vi "_main__.vi"() -> ()   [LabVIEW 2015]
doc: "Dialtek PKT-8 test programm"
uses:
  <vilib>/NI/Modbus Library/API/Master/Modbus Master.lvclass
  Load and Save Controls_LV2009.llb/RWC_Actions.ctl
  <vilib>/Utility/error.llb/DialogType.ctl
panel:
  out "Связь с блоком":bool
  in  "счетчик":u16
  in  "Tab Control":enum32{"Измерения", "Коэффициенты", "Настройки"}(tab)
  out "R8":dbl format="%.2f"
  out "R7":dbl format="%.2f"
  out "R6":dbl format="%.2f"
  out "R5":dbl format="%.2f"
  out "R4":dbl format="%.2f"
  out "R3":dbl format="%.2f"
  out "R2":dbl format="%.2f"
  out "R1":dbl format="%.2f"
  in  "8_ch_visible":bool=TRUE
  out "8":dbl format="%.2f"
  out "7":dbl format="%.2f"
  in  "7_ch_visible":bool=TRUE
  out "6":dbl format="%.2f"
  in  "6_ch_visible":bool=TRUE
  out "5":dbl format="%.2f"
  in  "5_ch_visible":bool=TRUE
  in  "4_ch_visible":bool=TRUE
  out "4":dbl format="%.2f"
  in  "3_ch_visible":bool=TRUE
  out "3":dbl format="%.2f"
  in  "2_ch_visible":bool=TRUE
  out "2":dbl format="%.2f"
  in  "1_ch_visible":bool=TRUE
  out "1":dbl format="%.2f"
  in  "xScale -":bool
  in  "xScale +":bool
  out "мин.":string="1"
  in  "Добавить время":dbl(ring)=300.0 items=["10 сек."=10.0, "1 мин."=60.0, "5 мин."=300.0, "20 мин."=1200.0]
  out "часы":string="0"
  out "сек.":string="0"
  in  "Coeff_cl_ch8":T1 caption="Канал 8" {"R" format="%#_16g"; "k7" format="%#_16g"; "k6" format="%#_16g"; "k5" format="%#_16g"; "k4" format="%#_16g"; "k3" format="%#_16g"; "k2" format="%#_16g"; "k1" format="%#_16g"}
  in  "Coeff_cl_ch7":T1 caption="Канал 7" {"R" format="%#_16g"; "k7" format="%#_16g"; "k6" format="%#_16g"; "k5" format="%#_16g"; "k4" format="%#_16g"; "k3" format="%#_16g"; "k2" format="%#_16g"; "k1" format="%#_16g"}
  in  "Coeff_cl_ch6":T1 caption="Канал 6" {"R" format="%#_16g"; "k7" format="%#_16g"; "k6" format="%#_16g"; "k5" format="%#_16g"; "k4" format="%#_16g"; "k3" format="%#_16g"; "k2" format="%#_16g"; "k1" format="%#_16g"}
  in  "Coeff_cl_ch5":T1 caption="Канал 5" {"R" format="%#_16g"; "k7" format="%#_16g"; "k6" format="%#_16g"; "k5" format="%#_16g"; "k4" format="%#_16g"; "k3" format="%#_16g"; "k2" format="%#_16g"; "k1" format="%#_16g"}
  in  "Coeff_cl_ch4":T1 caption="Канал 4" {"R" format="%#_16g"; "k7" format="%#_16g"; "k6" format="%#_16g"; "k5" format="%#_16g"; "k4" format="%#_16g"; "k3" format="%#_16g"; "k2" format="%#_16g"; "k1" format="%#_16g"}
  in  "Coeff_cl_ch3":T1 caption="Канал 3" {"R" format="%#_16g"; "k7" format="%#_16g"; "k6" format="%#_16g"; "k5" format="%#_16g"; "k4" format="%#_16g"; "k3" format="%#_16g"; "k2" format="%#_16g"; "k1" format="%#_16g"}
  in  "Coeff_cl_ch2":T1 caption="Канал 2" {"R" format="%#_16g"; "k7" format="%#_16g"; "k6" format="%#_16g"; "k5" format="%#_16g"; "k4" format="%#_16g"; "k3" format="%#_16g"; "k2" format="%#_16g"; "k1" format="%#_16g"}
  in  "Coeff_cl_ch1":T1 caption="Канал 1" {"R" format="%#_16g"; "k7" format="%#_16g"; "k6" format="%#_16g"; "k5" format="%#_16g"; "k4" format="%#_16g"; "k3" format="%#_16g"; "k2" format="%#_16g"; "k1" format="%#_16g"}
  in  "Сохранение в файл":bool=TRUE
  in  "интервал, сек.":u16=10 min=1 max=3600 step=1
  out "Path":string
  in  "buffer":u16=20 min=1 max=128
  in  "SPS":enum16{"2,5 SPS", "5 SPS", "10 SPS"}(ring)=enum."5 SPS"
  in  "ID":u8
  in  "Порт":u16
  in  "IP":string
  in  "Т min":dbl=4.0 min=-10.0 max=350.0 step=0.01
  in  "Т max":dbl=150.0 min=-10.0 max=150.0 step=0.01
  in  "Autoscale":bool=TRUE
  in  "Autoscale R":bool=TRUE
  in  "R max":dbl=150.0 min=-10.0 max=150.0 step=0.01
  in  "R min":dbl=4.0 min=-10.0 max=150.0 step=0.01
  out "refnum out":refnum<file>
  in  "stop":bool
  out "Сутки":string
  out "File header exist?":bool caption="Disconn"
  out "Graphs T":dynamicdata(graph) caption="T, K"
  out "Соед.":refnum<class "Modbus Master.lvclass">
  out "Graphs R":dynamicdata(graph) caption="R, Oм"
  # "№"
  # "T [ K ]"
  # "R [ Ohm ]"
  # ":"
  # ":"
  # "Настройки соединения"
  # "Настройки сохранения"
  # "Настройки АЦП"
  # "Буфер. усредн."
  # "Скорость изм."
  # "SPS = Samples Per Sec."
  # "Шкала Т"
  # "Шкала R"
types:
  T1 = cluster{"k1":ext, "k2":ext, "k3":ext, "k4":ext, "k5":ext, "k6":ext, "k7":ext, "R":ext}
  T2 = typedef "DialogType.ctl" = u16
  T3 = typedef "RWC_Actions.ctl" = enum16{"Read", "Write", "Read and Create"}
  T4 = typedef "LVDateTimeRec.ctl" = cluster{"fractional second":dbl, "second":i32, "minute":i32, "hour":i32, "day of month":i32, "month":i32, "year":i32, "day of week":i32, "day of year":i32, "DST":i32}
  T5 = cluster{"R1":dbl, "R2":dbl, "R3":dbl, "R4":dbl, "R5":dbl, "R6":dbl, "R7":dbl, "R8":dbl}
  T6 = cluster{"1":dbl, "2":dbl, "3":dbl, "4":dbl, "5":dbl, "6":dbl, "7":dbl, "8":dbl}
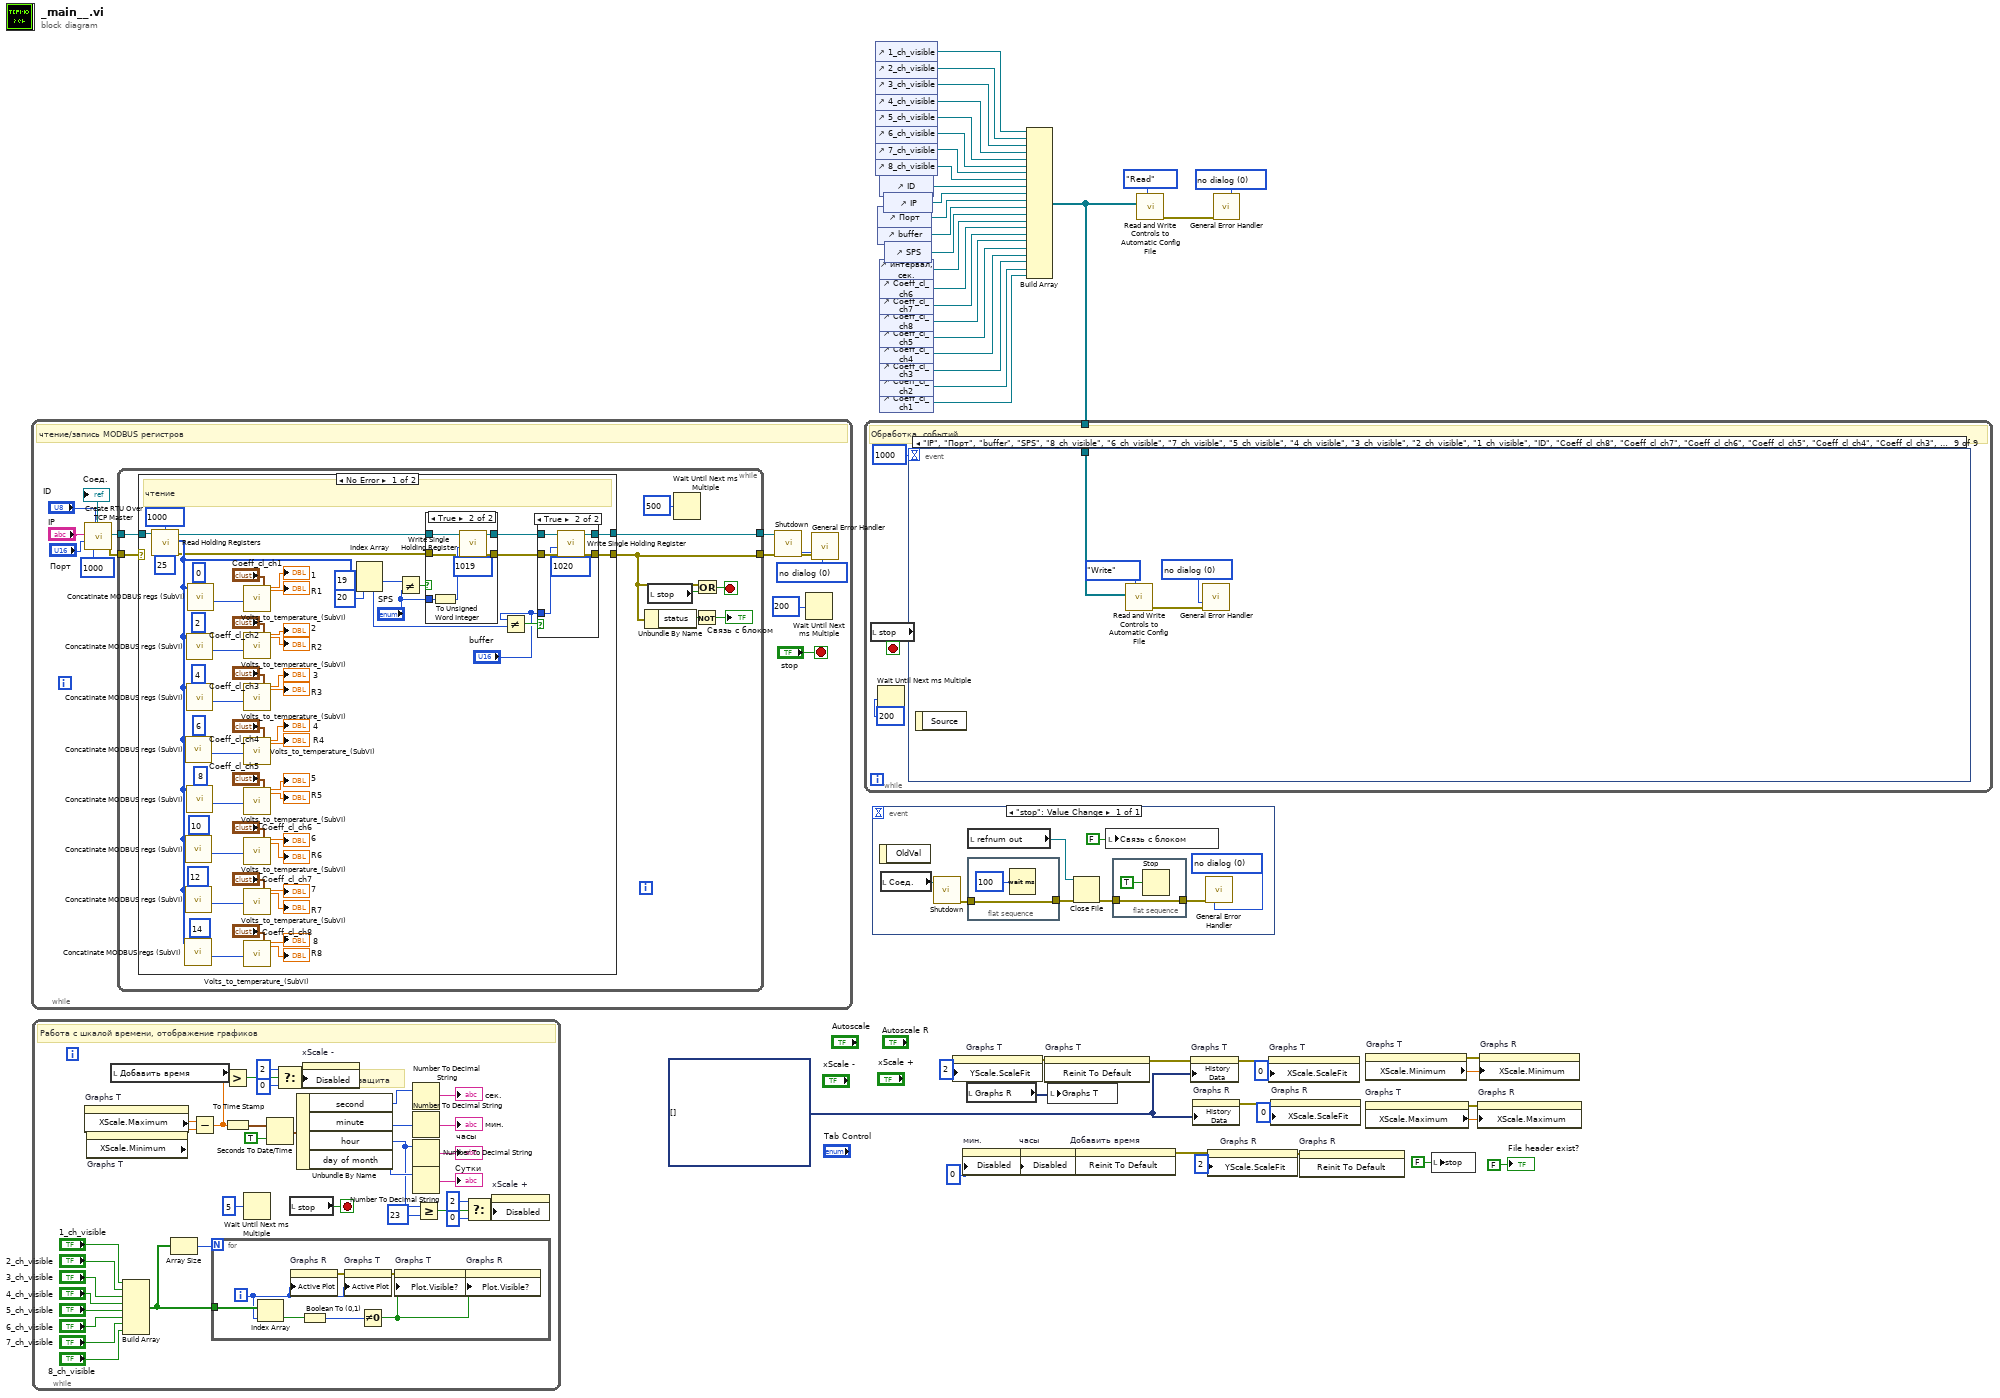
[diagram p0: block diagram]
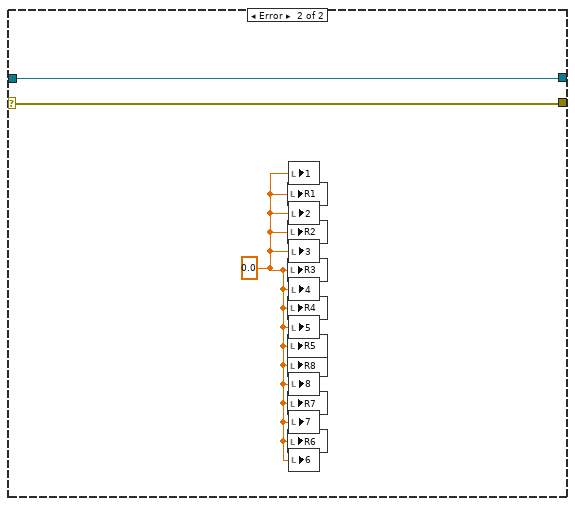
[diagram p4: hidden frame]
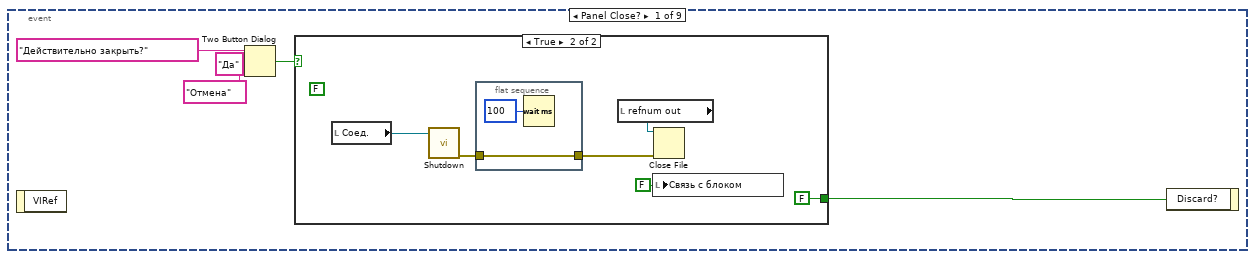
[diagram p5: hidden frame]
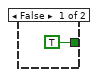
[diagram p6: hidden frame]
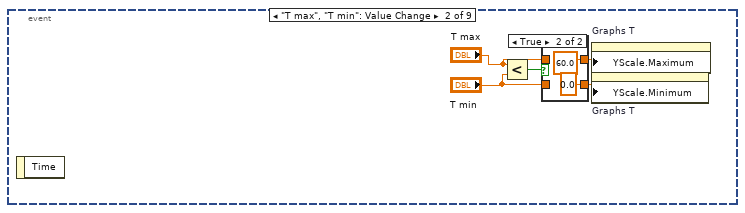
[diagram p7: hidden frame]
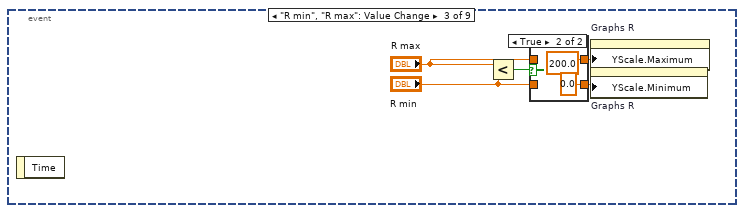
[diagram p9: hidden frame]
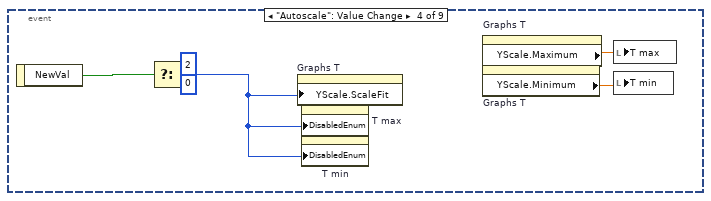
[diagram p11: hidden frame]
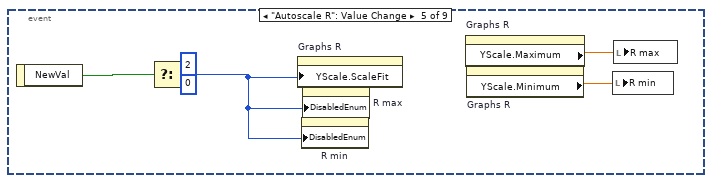
[diagram p12: hidden frame]
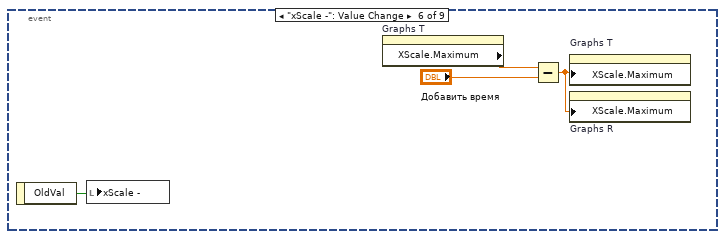
[diagram p13: hidden frame]
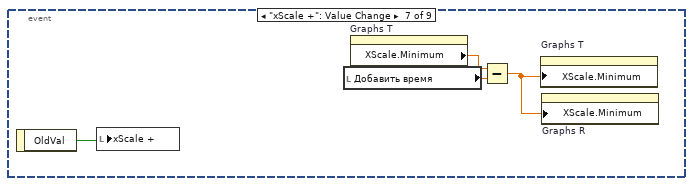
[diagram p14: hidden frame]
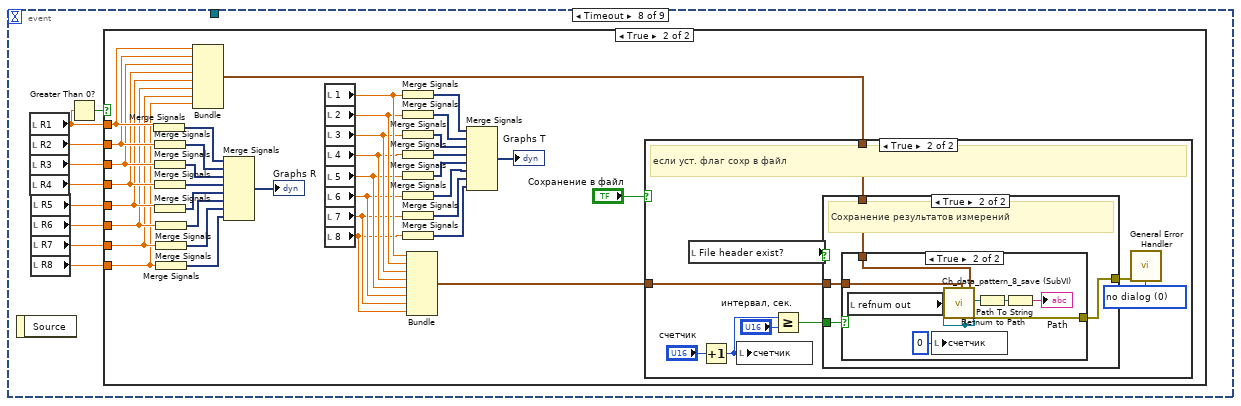
[diagram p15: hidden frame]
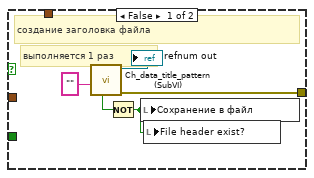
[diagram p18: hidden frame]
diagram:
  w13 = T2 0 items=["no dialog", "OK message", "continue or stop message", "OK message + warnings", "continue/stop + warnings"] ("type of dialog (OK msg:1)")
  w29 = dynamicdata[] [] ("History Data")
  w47 = u8 0 ("Disabled")
  n1 = while {
    stop <- "stop" stop-if-true
    w51 = T2 0 items=["no dialog", "OK message", "continue or stop message", "OK message + warnings", "continue/stop + warnings"] ("type of dialog (OK msg:1)")
    # "чтение/запись MODBUS регистров"
    n2 = call "Create RTU Over TCP Master.vi"("unit ID"="ID", "connect timeout ms"=1000, "port (502)"="Порт", "address"="IP") -> ("error out"=w55:errorcluster, "TCP master instance"=w56:refnum<class "Modbus Master.lvclass">)  [unwired: 6 in]
    "Соед." <- w56
    n3 = while {
      tunnel: w56 -> [w68]
      tunnel: w55 -> [w67]
      tunnel: [w61] -> w54
      tunnel: [w66] -> w53
      stop <- w64 stop-if-true
      n4 = case shown="No Error" w67 {
        selector: w67 -> [_ w145]
        tunnel: w68 -> [w124 w146]
        tunnel: [w103 w145] -> w61
        tunnel: [w104 w146] -> w66
        frame No Error {
          # "чтение"
          n5 = call-dynamic "Read Holding Registers.vi"("number of inputs"=u16 25, "starting address"=u16 1000, "Modbus master in"=w124) -> ("error out"=w102:errorcluster, "register values"=w106:u16[], "Modbus master out"=w107:refnum<class "Modbus Master.lvclass">)  [unwired: 6 in]
          n6 = call "Concatinate MODBUS regs (SubVI).vi"("LSB reg num"=u16 14, "registers array in"=w106) -> ("register data"=w81:i32)  [unwired: 8 in, 1 out]
          n7 = call "Concatinate MODBUS regs (SubVI).vi"("LSB reg num"=u16 6, "registers array in"=w106) -> ("register data"=w86:i32)  [unwired: 8 in, 1 out]
          n8 = call "Concatinate MODBUS regs (SubVI).vi"("LSB reg num"=u16 10, "registers array in"=w106) -> ("register data"=w83:i32)  [unwired: 8 in, 1 out]
          n9 = call "Concatinate MODBUS regs (SubVI).vi"("LSB reg num"=u16 12, "registers array in"=w106) -> ("register data"=w82:i32)  [unwired: 8 in, 1 out]
          n10 = call "Concatinate MODBUS regs (SubVI).vi"("LSB reg num"=u16 2, "registers array in"=w106) -> ("register data"=w95:i32)  [unwired: 8 in, 1 out]
          n11 = call "Concatinate MODBUS regs (SubVI).vi"("LSB reg num"=u16 4, "registers array in"=w106) -> ("register data"=w92:i32)  [unwired: 8 in, 1 out]
          n12 = call "Concatinate MODBUS regs (SubVI).vi"("LSB reg num"=u16 8, "registers array in"=w106) -> ("register data"=w84:i32)  [unwired: 8 in, 1 out]
          n13 = call "Concatinate MODBUS regs (SubVI).vi"("LSB reg num"=u16 0, "registers array in"=w106) -> ("register data"=w100:i32)  [unwired: 8 in, 1 out]
          n14 = call "Volts_to_temperature_(SubVI).vi"("input variable"=w100, "koeff. cluster"="Coeff_cl_ch1") -> ("T solvation"=→"1":dbl, "meas_voltage"=→"R1":dbl)  [unwired: 23 in, 1 out]
          n15 = call "Volts_to_temperature_(SubVI).vi"("input variable"=w95, "koeff. cluster"="Coeff_cl_ch2") -> ("T solvation"=→"2":dbl, "meas_voltage"=→"R2":dbl)  [unwired: 23 in, 1 out]
          n16 = call "Volts_to_temperature_(SubVI).vi"("input variable"=w92, "koeff. cluster"="Coeff_cl_ch3") -> ("T solvation"=→"3":dbl, "meas_voltage"=→"R3":dbl)  [unwired: 23 in, 1 out]
          n17 = call "Volts_to_temperature_(SubVI).vi"("input variable"=w86, "koeff. cluster"="Coeff_cl_ch4") -> ("T solvation"=→"4":dbl, "meas_voltage"=→"R4":dbl)  [unwired: 23 in, 1 out]
          n18 = call "Volts_to_temperature_(SubVI).vi"("input variable"=w84, "koeff. cluster"="Coeff_cl_ch5") -> ("T solvation"=→"5":dbl, "meas_voltage"=→"R5":dbl)  [unwired: 23 in, 1 out]
          n19 = call "Volts_to_temperature_(SubVI).vi"("input variable"=w83, "koeff. cluster"="Coeff_cl_ch6") -> ("T solvation"=→"6":dbl, "meas_voltage"=→"R6":dbl)  [unwired: 23 in, 1 out]
          n20 = call "Volts_to_temperature_(SubVI).vi"("input variable"=w82, "koeff. cluster"="Coeff_cl_ch7") -> ("T solvation"=→"7":dbl, "meas_voltage"=→"R7":dbl)  [unwired: 23 in, 1 out]
          n21 = call "Volts_to_temperature_(SubVI).vi"("input variable"=w81, "koeff. cluster"="Coeff_cl_ch8") -> ("T solvation"=→"8":dbl, "meas_voltage"=→"R8":dbl)  [unwired: 23 in, 1 out]
          n22 = Index Array(array=w106, index #1=19 ("index"), index #2=20 ("index")) -> (element #1=w110:u16, element #2=w115:u16)
          n23 = Not Equal?(x=w110, y="SPS") -> (x != y?=w111:bool)
          n24 = case shown="True" w111 {
            tunnel: w107 -> [w136 w143]
            tunnel: [w136 w141] -> w108
            tunnel: [w135 w140] -> w109
            tunnel: "SPS" -> [_ w138]
            tunnel: w102 -> [w135 w137]
            frame False {
            }
            frame True {
              n25 = To Unsigned Word Integer(number=w138) -> (unsigned 16bit integer=w139:u16)
              n26 = call-dynamic "Write Single Holding Register.vi"("error in"=w137, "register to write"=w139, "address"=u16 1019 ("starting address"), "Modbus master in"=w143) -> ("error out"=w140:errorcluster, "Modbus master out"=w141:refnum<class "Modbus Master.lvclass">)  [unwired: 6 in]
            }
          }
          n27 = Not Equal?(x="buffer", y=w115) -> (x != y?=w114:bool)
          n28 = case shown="True" w114 {
            tunnel: w108 -> [w128 w134]
            tunnel: w109 -> [w127 w133]
            tunnel: [w128 w131] -> w104
            tunnel: [w127 w130] -> w103
            tunnel: "buffer" -> [_ w129]
            frame False {
            }
            frame True {
              n29 = call-dynamic "Write Single Holding Register.vi"("error in"=w133, "register to write"=w129, "address"=u16 1020 ("starting address"), "Modbus master in"=w134) -> ("error out"=w130:errorcluster, "Modbus master out"=w131:refnum<class "Modbus Master.lvclass">)  [unwired: 6 in]
            }
          }
        }
        frame Error {
          w144 = 0.0 ("T1")
          n30 = local write "R1"(w144) -> ()
          n31 = local write "R2"(w144) -> ()
          n32 = local write "R3"(w144) -> ()
          n33 = local write "R4"(w144) -> ()
          n34 = local write "R5"(w144) -> ()
          n35 = local write "R8"(w144) -> ()
          n36 = local write "R7"(w144) -> ()
          n37 = local write "R6"(w144) -> ()
          n38 = local write "1"(w144) -> ()
          n39 = local write "2"(w144) -> ()
          n40 = local write "3"(w144) -> ()
          n41 = local write "4"(w144) -> ()
          n42 = local write "5"(w144) -> ()
          n43 = local write "8"(w144) -> ()
          n44 = local write "7"(w144) -> ()
          n45 = local write "6"(w144) -> ()
        }
      }
      n46 = Unbundle By Name(w61) -> ("status"=w63:bool)
      n47 = local read "stop"() -> (w65:bool)
      n48 = Wait Until Next ms Multiple(millisecond multiple=u32 500) -> ()  [unwired: 1 out]
      n49 = Not(x=w63) -> (.not. x?=→"Связь с блоком":bool)
      n50 = Or(x=w61, y=w65) -> (x .or. y?=w64:bool)
    }
    n51 = call-dynamic "Shutdown.vi"("error in"=w54, "Modbus master in"=w53) -> ("error out"=w52:errorcluster)  [unwired: 9 in]
    n52 = Wait Until Next ms Multiple(millisecond multiple=u32 200) -> ()  [unwired: 1 out]
    n53 = call <vilib>:"General Error Handler.vi"("type of dialog (OK msg:1)"=w51, "error in (no error)"=w52) -> ()  [unwired: 1 in, 13 out]
  }
  n54 = while {
    stop <- w182 stop-if-true
    # "защита"
    # "Работа с шкалой времени, отображение графиков"
    n55 = property on="Graphs T" class="WFChart (strict)"() -> ("XScale.Maximum"=w158:dbl)  [unwired: 2 in, 2 out]
    n56 = property on="Graphs T" class="WFChart (strict)"() -> ("XScale.Minimum"=w157:dbl)  [unwired: 2 in, 2 out]
    n57 = local read "Добавить время"() -> (w181:dbl)
    n58 = Build Array("1_ch_visible", "2_ch_visible", "3_ch_visible", "4_ch_visible", "5_ch_visible", "6_ch_visible", "7_ch_visible", "8_ch_visible") -> (w147:bool[])
    n59 = Array Size(array=w147) -> (size(s)=w148:i32)
    n60 = Subtract(x=w158, y=w157) -> (x-y=w171:dbl)
    n61 = for {
      N: w148 -> [_]
      tunnel: w147 -> [w190]
      i -> [w187]
      n62 = Index Array(array=w190, index=w187) -> (element=w189:bool)
      n63 = property on="Graphs R" class="WFChart (strict)"("Active Plot"=w187) -> (error out=w183:errorcluster)  [unwired: 2 in, 1 out]
      n64 = Boolean To (0,1)(Boolean=w189) -> (0, 1=w188:i16)
      n65 = property on="Graphs T" class="WFChart (strict)"(error in=w183, "Active Plot"=w187) -> (error out=w184:errorcluster)  [unwired: 1 in, 1 out]
      n66 = Not Equal To 0?(x=w188) -> (x != 0?=w186:bool)
      n67 = property on="Graphs T" class="WFChart (strict)"(error in=w184, "Plot.Visible?"=w186) -> (error out=w185:errorcluster)  [unwired: 1 in, 1 out]
      n68 = property on="Graphs R" class="WFChart (strict)"(error in=w185, "Plot.Visible?"=w186) -> ()  [unwired: 1 in, 2 out]
    }
    n69 = Greater?(x=w181, y=w171) -> (0:w164:bool)
    n70 = To Time Stamp(1:w171) -> (0:w179:timestamp)
    n71 = Wait Until Next ms Multiple(millisecond multiple=u32 5) -> ()  [unwired: 1 out]
    n72 = Seconds To Date/Time(time stamp (now)=w179, to UTC (F)=TRUE) -> (date time rec=w178:T4)
    n73 = Select(t=u8 2 ("Disabled"), s=w164, f=u8 0 ("Disabled")) -> (s? t:f=w167:u8)
    n74 = local read "stop"() -> (w182:bool)
    n75 = Unbundle By Name(w178) -> ("second"=w177:i32, "minute"=w176:i32, "hour"=w169:i32, "day of month"=w175:i32)
    n76 = property on="xScale -" class="Bool (strict)"("Disabled"=w167) -> ()  [unwired: 2 in, 2 out]
    n77 = Number To Decimal String(number=w177) -> (decimal integer string=→"сек.":string)  [unwired: 1 out]
    n78 = Number To Decimal String(number=w176) -> (decimal integer string=→"мин.":string)  [unwired: 1 out]
    n79 = Number To Decimal String(number=w169) -> (decimal integer string=→"часы":string)  [unwired: 1 out]
    n80 = Number To Decimal String(number=w175) -> (decimal integer string=→"Сутки":string)  [unwired: 1 out]
    n81 = Greater Or Equal?(x=w169, y=23) -> (x >= y?=w160:bool)
    n82 = Select(t=u8 2 ("Disabled"), s=w160, f=u8 0 ("Disabled")) -> (s? t:f=w163:u8)
    n83 = property on="xScale +" class="Bool (strict)"("Disabled"=w163) -> ()  [unwired: 2 in, 2 out]
  }
  n84 = event shown="[0] \"stop\": Value Change" {
    selector: _ -> [_]
    dyn-events: _ -> [_]
    timeout: _ -> [_]
    event "stop": Value Change {
      w195 = T2 0 items=["no dialog", "OK message", "continue or stop message", "OK message + warnings", "continue/stop + warnings"] ("type of dialog (OK msg:1)")
      n85 = event-data() -> ()  [unwired: 1 in, 1 out]
      n86 = local read "Соед."() -> (w197:refnum<class "Modbus Master.lvclass">)
      n87 = call-dynamic "Shutdown.vi"("Modbus master in"=w197) -> ("error out"=w196:errorcluster)  [unwired: 10 in]
      n88 = local read "refnum out"() -> (w198:refnum<file>)
      n89 = flat-sequence {
        tunnel: w196 -> [w201]
        tunnel: [w201] -> w194
        frame #0 {
          n90 = Wait (ms)(milliseconds to wait=u32 100) -> ()  [unwired: 1 out]
        }
      }
      n91 = Close File(refnum=w198, error in=w194) -> (error out=w192:errorcluster)  [unwired: 1 out]
      n92 = local write "Связь с блоком"(FALSE ("Запись в файл")) -> ()
      n93 = flat-sequence {
        tunnel: [w199] -> w191
        tunnel: w192 -> [w199]
        frame #0 {
          n94 = Stop(stop? (T)=TRUE) -> ()
        }
      }
      n95 = call <vilib>:"General Error Handler.vi"("error in (no error)"=w191, "[exception action] (none:0)"=w195) -> ()  [unwired: 2 in, 12 out]
    }
  }
  n96 = control-ref of="1_ch_visible"() -> (w26:refnum<vi>)
  n97 = control-ref of="2_ch_visible"() -> (w25:refnum<vi>)
  n98 = control-ref of="3_ch_visible"() -> (w24:refnum<vi>)
  n99 = control-ref of="4_ch_visible"() -> (w23:refnum<vi>)
  n100 = control-ref of="5_ch_visible"() -> (w22:refnum<vi>)
  n101 = control-ref of="6_ch_visible"() -> (w21:refnum<vi>)
  n102 = control-ref of="7_ch_visible"() -> (w20:refnum<vi>)
  n103 = control-ref of="8_ch_visible"() -> (w19:refnum<vi>)
  n104 = control-ref of="Порт"() -> (w11:refnum<vi>)
  n105 = control-ref of="buffer"() -> (w10:refnum<vi>)
  n106 = control-ref of="ID"() -> (w18:refnum<vi>)
  n107 = control-ref of="интервал, сек."() -> (w9:refnum<vi>)
  n108 = control-ref of="Coeff_cl_ch6"() -> (w8:refnum<vi>)
  n109 = control-ref of="Coeff_cl_ch7"() -> (w7:refnum<vi>)
  n110 = control-ref of="Coeff_cl_ch8"() -> (w6:refnum<vi>)
  n111 = control-ref of="Coeff_cl_ch5"() -> (w5:refnum<vi>)
  n112 = control-ref of="Coeff_cl_ch4"() -> (w4:refnum<vi>)
  n113 = control-ref of="Coeff_cl_ch3"() -> (w3:refnum<vi>)
  n114 = control-ref of="Coeff_cl_ch2"() -> (w2:refnum<vi>)
  n115 = control-ref of="Coeff_cl_ch1"() -> (w1:refnum<vi>)
  n116 = control-ref of="IP"() -> (w17:refnum<vi>)
  n117 = control-ref of="SPS"() -> (w16:refnum<vi>)
  n118 = property on="Graphs T" class="WFChart (strict)"("YScale.ScaleFit"=u8 2 ("Y Scale.Scale Fit")) -> (error out=w38:errorcluster)  [unwired: 2 in, 1 out]
  n119 = property on="мин." class="Str"("Disabled"=w47) -> (error out=w46:errorcluster)  [unwired: 2 in, 1 out]
  n120 = local read "Graphs R"() -> (w28:dynamicdata)
  n121 = property on="часы" class="Str"(error in=w46, "Disabled"=w47) -> (error out=w45:errorcluster)  [unwired: 1 in, 1 out]
  n122 = Build Array(w26, w25, w24, w23, w22, w21, w20, w19, w18, w17, w11, w10, w16, w9, w8, w7, w6, w5, w4, w3, w2, w1) -> (w12:refnum<vi>[])
  n123 = while {
    tunnel: w12 -> [w203]
    stop <- w205 stop-if-true
    # "Обработка  событий"
    n124 = local read "stop"() -> (w205:bool)
    n125 = Wait Until Next ms Multiple(millisecond multiple=u32 200) -> ()  [unwired: 1 out]
    n126 = event shown="[8] \"IP\", \"Порт\", \"buffer\", \"SPS\", \"8_ch_visible\", \"6_ch_visible\", \"7_ch_visible\", \"5_ch_visible\", \"4_ch_visible\", \"3_ch_visible\", \"2_ch_visible\", \"1_ch_visible\", \"ID\", \"Coeff_cl_ch8\", \"Coeff_cl_ch7\", \"Coeff_cl_ch6\", \"Coeff_cl_ch5\", \"Coeff_cl_ch4\", \"Coeff_cl_ch3\", \"Coeff_cl_ch2\", \"Coeff_cl_ch1\": Value Change" {
      selector: _ -> [_ _ _ _ _ _ _ _ _]
      dyn-events: _ -> [_ _ _ _ _ _ _ _ _]
      timeout: 1000 -> [_ _ _ _ _ _ _ _ _]
      tunnel: w203 -> [_ _ _ _ _ _ _ _ w333]
      event Panel Close? {
        n127 = event-data() -> ()  [unwired: 2 out]
        n128 = Two Button Dialog(message="Действительно закрыть?", 1:"Отмена" ("T button name (\"OK\")"), 2:"Да" ("T button name (\"OK\")")) -> (T button?=w211:bool)
        n129 = case shown="True" w211 {
          tunnel: [TRUE ("Discard?") FALSE ("Discard?")] -> w207
          frame False {
          }
          frame True {
            (unwired) FALSE ("Запись в файл")
            n130 = local read "Соед."() -> (w217:refnum<class "Modbus Master.lvclass">)
            n131 = call-dynamic "Shutdown.vi"("Modbus master in"=w217) -> ("error out"=w216:errorcluster)  [unwired: 10 in]
            n132 = flat-sequence {
              tunnel: w216 -> [w219]
              tunnel: [w219] -> w215
              frame #0 {
                n133 = Wait (ms)(milliseconds to wait=u32 100) -> ()  [unwired: 1 out]
              }
            }
            n134 = local read "refnum out"() -> (w213:refnum<file>)
            n135 = local write "Связь с блоком"(FALSE ("Связь с блоком 4")) -> ()
            n136 = Close File(refnum=w213, error in=w215) -> ()  [unwired: 2 out]
          }
        }
        n137 = event-data("Discard?"=w207) -> ()  [unwired: 1 in, 1 out]
      }
      event "Т max", "Т min": Value Change {
        n138 = event-data() -> ()  [unwired: 2 out]
        n139 = Less?(x="Т max", y="Т min") -> (x < y?=w225:bool)
        n140 = case shown="True" w225 {
          tunnel: [w226 60.0 ("x+1")] -> w223
          tunnel: [w227 0.0 ("x+1")] -> w224
          tunnel: "Т max" -> [w226 _]
          tunnel: "Т min" -> [w227 _]
          frame False {
          }
          frame True {
          }
        }
        n141 = property on="Graphs T" class="WFChart (strict)"("YScale.Maximum"=w223) -> ()  [unwired: 2 in, 2 out]
        n142 = property on="Graphs T" class="WFChart (strict)"("YScale.Minimum"=w224) -> ()  [unwired: 2 in, 2 out]
      }
      event "R min", "R max": Value Change {
        n143 = event-data() -> ()  [unwired: 2 out]
        n144 = Less?(x="R max", y="R min") -> (x < y?=w234:bool)
        n145 = case shown="True" w234 {
          tunnel: [w235 200.0 ("x+1")] -> w233
          tunnel: [w236 0.0 ("x+1")] -> w232
          tunnel: "R max" -> [w235 _]
          tunnel: "R min" -> [w236 _]
          frame False {
          }
          frame True {
          }
        }
        n146 = property on="Graphs R" class="WFChart (strict)"("YScale.Maximum"=w233) -> ()  [unwired: 2 in, 2 out]
        n147 = property on="Graphs R" class="WFChart (strict)"("YScale.Minimum"=w232) -> ()  [unwired: 2 in, 2 out]
      }
      event "Autoscale": Value Change {
        n148 = event-data() -> ("NewVal"=w239:bool)  [unwired: 1 out]
        n149 = Select(t=u8 2 ("Y Scale.Scale Fit"), s=w239, f=u8 0 ("Y Scale.Scale Fit")) -> (s? t:f=w242:u8)
        n150 = property on="Graphs T" class="WFChart (strict)"("YScale.ScaleFit"=w242) -> ()  [unwired: 2 in, 2 out]
        n151 = property on="Т max" class="DigNum (strict)"("DisabledEnum"=w242) -> ()  [unwired: 2 in, 2 out]
        n152 = property on="Т min" class="DigNum (strict)"("DisabledEnum"=w242) -> ()  [unwired: 2 in, 2 out]
        n153 = property on="Graphs T" class="WFChart (strict)"() -> ("YScale.Maximum"=w244:dbl)  [unwired: 2 in, 2 out]
        n154 = property on="Graphs T" class="WFChart (strict)"() -> ("YScale.Minimum"=w243:dbl)  [unwired: 2 in, 2 out]
        n155 = local write "Т max"(w244) -> ()
        n156 = local write "Т min"(w243) -> ()
      }
      event "Autoscale R": Value Change {
        n157 = event-data() -> ("NewVal"=w248:bool)  [unwired: 1 out]
        n158 = Select(t=u8 2 ("Y Scale.Scale Fit"), s=w248, f=u8 0 ("Y Scale.Scale Fit")) -> (s? t:f=w245:u8)
        n159 = property on="Graphs R" class="WFChart (strict)"("YScale.ScaleFit"=w245) -> ()  [unwired: 2 in, 2 out]
        n160 = property on="R min" class="DigNum (strict)"("DisabledEnum"=w245) -> ()  [unwired: 2 in, 2 out]
        n161 = property on="R max" class="DigNum (strict)"("DisabledEnum"=w245) -> ()  [unwired: 2 in, 2 out]
        n162 = property on="Graphs R" class="WFChart (strict)"() -> ("YScale.Maximum"=w247:dbl)  [unwired: 2 in, 2 out]
        n163 = property on="Graphs R" class="WFChart (strict)"() -> ("YScale.Minimum"=w246:dbl)  [unwired: 2 in, 2 out]
        n164 = local write "R min"(w246) -> ()
        n165 = local write "R max"(w247) -> ()
      }
      event "xScale -": Value Change {
        n166 = event-data() -> ("OldVal"=w254:bool)  [unwired: 1 out]
        n167 = local write "xScale -"(w254) -> ()
        n168 = property on="Graphs T" class="WFChart (strict)"() -> ("XScale.Maximum"=w252:dbl)  [unwired: 2 in, 2 out]
        n169 = Subtract(x=w252, y="Добавить время") -> (x-y=w251:dbl)
        n170 = property on="Graphs T" class="WFChart (strict)"("XScale.Maximum"=w251) -> ()  [unwired: 2 in, 2 out]
        n171 = property on="Graphs R" class="WFChart (strict)"("XScale.Maximum"=w251) -> ()  [unwired: 2 in, 2 out]
      }
      event "xScale +": Value Change {
        n172 = event-data() -> ("OldVal"=w258:bool)  [unwired: 1 out]
        n173 = local write "xScale +"(w258) -> ()
        n174 = local read "Добавить время"() -> (w257:dbl)
        n175 = property on="Graphs T" class="WFChart (strict)"() -> ("XScale.Minimum"=w256:dbl)  [unwired: 2 in, 2 out]
        n176 = Subtract(x=w256, y=w257) -> (x-y=w255:dbl)
        n177 = property on="Graphs T" class="WFChart (strict)"("XScale.Minimum"=w255) -> ()  [unwired: 2 in, 2 out]
        n178 = property on="Graphs R" class="WFChart (strict)"("XScale.Minimum"=w255) -> ()  [unwired: 2 in, 2 out]
      }
      event Timeout {
        n179 = event-data() -> ()  [unwired: 2 out]
        n180 = local read "R1"() -> (w260:dbl)
        n181 = local read "R2"() -> (w267:dbl)
        n182 = local read "R3"() -> (w266:dbl)
        n183 = local read "R4"() -> (w265:dbl)
        n184 = local read "R5"() -> (w261:dbl)
        n185 = local read "R6"() -> (w262:dbl)
        n186 = local read "R7"() -> (w263:dbl)
        n187 = local read "R8"() -> (w264:dbl)
        n188 = Greater Than 0?(x=w260) -> (x > 0?=w259:bool)
        n189 = case shown="True" w259 {
          tunnel: w267 -> [_ w285]
          tunnel: w266 -> [_ w284]
          tunnel: w265 -> [_ w283]
          tunnel: w264 -> [_ w279]
          tunnel: w263 -> [_ w280]
          tunnel: w262 -> [_ w281]
          tunnel: w261 -> [_ w282]
          tunnel: w260 -> [_ w286]
          frame False {
          }
          frame True {
            n190 = Merge Signals(w286) -> (w298:dynamicdata)
            n191 = Merge Signals(w285) -> (w299:dynamicdata)
            n192 = Merge Signals(w284) -> (w297:dynamicdata)
            n193 = Merge Signals(w283) -> (w295:dynamicdata)
            n194 = Merge Signals(w282) -> (w290:dynamicdata)
            n195 = Merge Signals(w281) -> (w289:dynamicdata)
            n196 = Merge Signals(w280) -> (w288:dynamicdata)
            n197 = Merge Signals(w279) -> (w287:dynamicdata)
            n198 = Bundle("R1"=w286, "R2"=w285, "R3"=w284, "R4"=w283, "R5"=w282, "R6"=w281, "R7"=w280, "R8"=w279) -> (w278:T5)  [unwired: 1 in]
            n199 = Merge Signals(w298, w299, w297, w295, w290, w289, w288, w287) -> (→"Graphs R":dynamicdata)
            n200 = local read "1"() -> (w277:dbl)
            n201 = local read "2"() -> (w276:dbl)
            n202 = local read "3"() -> (w275:dbl)
            n203 = local read "4"() -> (w274:dbl)
            n204 = local read "5"() -> (w273:dbl)
            n205 = local read "6"() -> (w272:dbl)
            n206 = local read "7"() -> (w271:dbl)
            n207 = local read "8"() -> (w270:dbl)
            n208 = Merge Signals(w277) -> (w304:dynamicdata)
            n209 = Merge Signals(w276) -> (w303:dynamicdata)
            n210 = Merge Signals(w275) -> (w302:dynamicdata)
            n211 = Merge Signals(w274) -> (w301:dynamicdata)
            n212 = Merge Signals(w273) -> (w294:dynamicdata)
            n213 = Merge Signals(w272) -> (w293:dynamicdata)
            n214 = Merge Signals(w271) -> (w292:dynamicdata)
            n215 = Merge Signals(w270) -> (w291:dynamicdata)
            n216 = Bundle("1"=w277, "2"=w276, "3"=w275, "4"=w274, "5"=w273, "6"=w272, "7"=w271, "8"=w270) -> (w269:T6)  [unwired: 1 in]
            n217 = Merge Signals(w304, w303, w302, w301, w294, w293, w292, w291) -> (→"Graphs T":dynamicdata)
            n218 = case shown="True" "Сохранение в файл" {
              tunnel: w278 -> [_ w306]
              tunnel: w269 -> [_ w305]
              frame False {
              }
              frame True {
                w313 = T2 0 items=["no dialog", "OK message", "continue or stop message", "OK message + warnings", "continue/stop + warnings"] ("type of dialog (OK msg:1)")
                # "если уст. флаг сохр в файл"
                n219 = local read "File header exist?"() -> (w308:bool)
                n220 = Increment(x="счетчик") -> (x+1=w310:u16)
                n221 = local write "счетчик"(w310) -> ()
                n222 = Greater Or Equal?(x=w310, y="интервал, сек.") -> (x >= y?=w309:bool)
                n223 = case shown="True" w308 {
                  tunnel: [w316 w321] -> w312
                  tunnel: w309 -> [_ w322]
                  tunnel: w306 -> [_ w320]
                  tunnel: w305 -> [_ w319]
                  frame False {
                    # "выполняется 1 раз"
                    # "создание заголовка файла"
                    n224 = call "Ch_data_title_pattern (SubVI).vi"("Единица измерений"="") -> ("error out"=w316:errorcluster, "Byte Stream File out"=→"refnum out":refnum<file>, "cancelled"=w315:bool)  [unwired: 7 in, 1 out]
                    n225 = Not(x=w315) -> (.not. x?=w314:bool)
                    n226 = local write "Сохранение в файл"(w314) -> ()
                    n227 = local write "File header exist?"(w314) -> ()
                  }
                  frame True {
                    # "Сохранение результатов измерений"
                    n228 = case shown="True" w322 {
                      tunnel: [_ w326] -> w321
                      tunnel: w320 -> [_ w325]
                      tunnel: w319 -> [_ w324]
                      frame False {
                      }
                      frame True {
                        n229 = local read "refnum out"() -> (w323:refnum<file>)
                        n230 = local write "счетчик"(u8 0 ("счетчик")) -> ()
                        n231 = call "Ch_data_pattern_8_save (SubVI).vi"("T Cluster"=w324, "file"=w323, "R cluster"=w325) -> ("error out"=w326:errorcluster)  [unwired: 24 in]
                        n232 = Refnum to Path(1:w323) -> (0:w329:path)
                        n233 = Path To String(path=w329) -> (string=→"Path":string)
                      }
                    }
                  }
                }
                n234 = call <vilib>:"General Error Handler.vi"("type of dialog (OK msg:1)"=w313, "error in (no error)"=w312) -> ()  [unwired: 1 in, 13 out]
              }
            }
          }
        }
      }
      event "IP", "Порт", "buffer", "SPS", "8_ch_visible", "6_ch_visible", "7_ch_visible", "5_ch_visible", "4_ch_visible", "3_ch_visible", "2_ch_visible", "1_ch_visible", "ID", "Coeff_cl_ch8", "Coeff_cl_ch7", "Coeff_cl_ch6", "Coeff_cl_ch5", "Coeff_cl_ch4", "Coeff_cl_ch3", "Coeff_cl_ch2", "Coeff_cl_ch1": Value Change {
        w330 = T2 0 items=["no dialog", "OK message", "continue or stop message", "OK message + warnings", "continue/stop + warnings"] ("type of dialog (OK msg:1)")
        n235 = event-data() -> ()  [unwired: 2 out]
        n236 = call "Read and Write Controls to Automatic Config File.vi"("Action"=RWC_Actions."Write", "Control References"=w333) -> ("error out"=w331:errorcluster)  [unwired: 9 in]
        n237 = call <vilib>:"General Error Handler.vi"("type of dialog (OK msg:1)"=w330, "error in (no error)"=w331) -> ()  [unwired: 1 in, 13 out]
      }
    }
  }
  n238 = invoke on="Graphs T" class="WFChart (strict)" method="Reinit To Default"(error in=w38) -> (error out=w30:errorcluster)  [unwired: 2 in, 2 out]
  n239 = local write "Graphs T"(w28) -> ()
  n240 = invoke on="Добавить время" class="Ring (strict)" method="Reinit To Default"(error in=w45) -> (error out=w27:errorcluster)  [unwired: 2 in, 2 out]
  n241 = call "Read and Write Controls to Automatic Config File.vi"("Action"=RWC_Actions."Read", "Control References"=w12) -> ("error out"=w14:errorcluster)  [unwired: 9 in]
  n242 = property on="Graphs T" class="WFChart (strict)"(error in=w30, "History Data"=w29) -> (error out=w35:errorcluster)  [unwired: 1 in, 1 out]
  n243 = property on="Graphs R" class="WFChart (strict)"("History Data"=w29) -> (error out=w44:errorcluster)  [unwired: 2 in, 1 out]
  n244 = property on="Graphs R" class="WFChart (strict)"(error in=w27, "YScale.ScaleFit"=u8 2 ("Y Scale.Scale Fit")) -> (error out=w39:errorcluster)  [unwired: 1 in, 1 out]
  n245 = call <vilib>:"General Error Handler.vi"("type of dialog (OK msg:1)"=w13, "error in (no error)"=w14) -> ()  [unwired: 1 in, 13 out]
  n246 = property on="Graphs T" class="WFChart (strict)"(error in=w35, "XScale.ScaleFit"=u8 0 ("Y Scale.Scale Fit")) -> ()  [unwired: 1 in, 2 out]
  n247 = property on="Graphs R" class="WFChart (strict)"(error in=w44, "XScale.ScaleFit"=u8 0 ("Y Scale.Scale Fit")) -> ()  [unwired: 1 in, 2 out]
  n248 = invoke on="Graphs R" class="WFChart (strict)" method="Reinit To Default"(error in=w39) -> ()  [unwired: 2 in, 3 out]
  n249 = property on="Graphs T" class="WFChart (strict)"() -> (error out=w31:errorcluster, "XScale.Maximum"=w32:dbl)  [unwired: 2 in, 1 out]
  n250 = property on="Graphs T" class="WFChart (strict)"() -> (error out=w33:errorcluster, "XScale.Minimum"=w34:dbl)  [unwired: 2 in, 1 out]
  n251 = local write "stop"(FALSE ("Boolean")) -> ()
  n252 = property on="Graphs R" class="WFChart (strict)"(error in=w31, "XScale.Maximum"=w32) -> ()  [unwired: 1 in, 2 out]
  n253 = property on="Graphs R" class="WFChart (strict)"(error in=w33, "XScale.Minimum"=w34) -> ()  [unwired: 1 in, 2 out]
  "File header exist?" <- FALSE ("flag1")
